vi "Configuration Utility.vi"() -> ()   [LabVIEW 2013, in "configuration library.lvlib"]
doc: "This is the main VI for the configuration editor."
uses:
  configuration library.lvlib
  Controls/StateCluster.ctl
  <vilib>/NI/Tag Bus Data Framework/Configuration Editor/Classes/SystemConfigRepo/SystemConfigRepo.lvclass
  <vilib>/CEF_TreeControl/Node/NodeRef.ctl
  <vilib>/CEF_TreeControl/Node/NISE_CEF_Node.lvclass
  <vilib>/CEF_TreeControl/Node/UserEventRef.ctl
  <vilib>/CEF_TreeControl/Controls/EventCluster.ctl
  subVI/SplashScreen/splash screen.ctl
  subVI/SplashScreen/notifier data.ctl
  Controls/add message.ctl
  Controls/MoveMessage.ctl
  <vilib>/NI/Tag Bus Module Framework/plugin discovery singleton/class discovery singleton methods.ctl
  <vilib>/NI/Tag Bus Data Framework/Configuration Editor/Classes/Systems/Systems.lvclass
  <vilib>/NI/Tag Bus Data Framework/Framework Configuration Classes/platypus configuration/systems cluster.ctl
  <vilib>/NI/Tag Bus Data Framework/Framework Configuration Classes/system configuration/PL_System Configuration.lvclass
  <vilib>/NI/Tag Bus Data Framework/Framework Configuration Classes/platypus configuration/targets cluster.ctl
  <vilib>/NI/Tag Bus Data Framework/Framework Configuration Classes/target configuration/PL_Target Configuration.lvclass
  <vilib>/NI/Tag Bus Data Framework/Framework Configuration Classes/platypus configuration/engines cluster.ctl
  <vilib>/NI/Module Execution Interface/Engine Configuration/engine configuration.lvclass
  <vilib>/NI/Tag Bus Module Framework/module configuration/TBM module configuration.lvclass
  <vilib>/NI/Tag Bus Data Framework/Configuration Editor/Classes/SystemConfigRepo/SystemConfigRepo.lvclass/SystemConfigRepo.ctl
  <vilib>/CEF_TreeControl/Repository/NISE_CEF_Repository.lvclass
  <vilib>/NI/AMC/Create Single Message.vi
  <vilib>/NI/AMC/Update Message Routing Info.vi
  <vilib>/NI/AMC/Read Termination Message.vi
  <vilib>/NI/Tag Bus Data Framework/Configuration Editor/subVIs/Glyphs Status.ctl
  <vilib>/NI/Tag Bus Data Framework/Configuration Editor/subVIs/Add status to name.vi
  <vilib>/NI/AMC/Send Message.vi
  <vilib>/NI/AMC/Globals.vi
  <vilib>/NI/Tag Bus Data Framework/Configuration Editor/Classes/Module editor node/module editor node.lvclass
  <vilib>/NI/Tag Bus Data Framework/Configuration Editor/Classes/EngineTags/EngineTags.lvclass
  <vilib>/NI/Module Timing Source/timing source/TBM timing source.lvclass
  <vilib>/NI/Tag Bus Data Framework/Configuration Editor/Classes/TBM Configuration Node/TBM Configuration Node.lvclass
  <vilib>/NI/Tag Bus Module Framework/root configuration/TBM configuration.lvclass
  <vilib>/NI/Tag Bus Data Framework/Configuration Editor/Classes/Targets/Targets.lvclass
  <vilib>/NI/Tag Bus Data Framework/Configuration Editor/Classes/Engine Parent/Engine Parent Editor Node.lvclass
  <vilib>/NI/Tag Bus Module Framework/channel/TBM channel.lvclass
  <vilib>/NI/AMC/AMC.lvlib
  <vilib>/CEF_TreeControl/NISE_CEF_TreeControl.lvlib
  subVI/SplashScreen/splash screen.lvlib
  <vilib>/NI/Tag Bus Data Framework/Framework Configuration Classes/class cache/PL_class cache.lvlib
  <vilib>/NI/Tag Bus Module Framework/plugin discovery singleton/class discovery singleton.lvlib
  <vilib>/NI/Tag Bus Data Framework/Configuration Editor/PL Framework Configuration Tool.lvlib
  <vilib>/NI/Tag Bus Data Framework/Framework Configuration Classes/platypus configuration/PLConfigurationSerializer.lvlib
panel:
  in  "Exit":bool
  in  "View":string(tree)
  # "Tag Bus Configuration Editor"
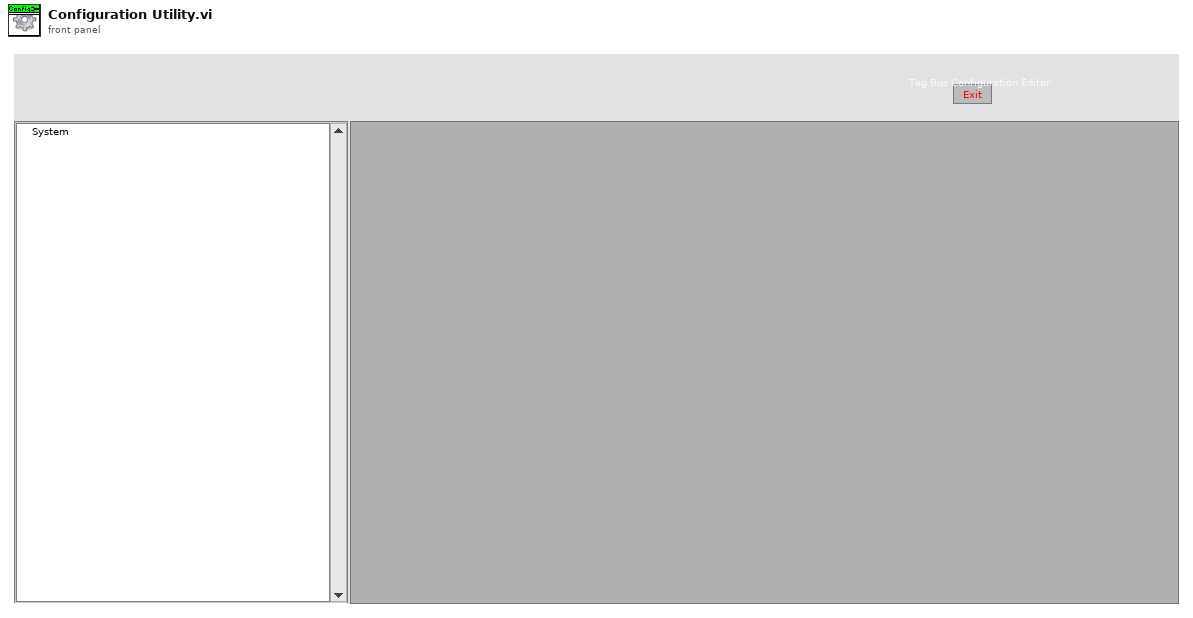
[diagram p1: front panel]
types:
  T1 = enum32{"Invalid", "Standard", "Closed", "Hidden", "Minimized", "Maximized"}
  T2 = typedef "configuration library.lvlib/StateCluster.ctl" = cluster{"repository":refnum<class "SystemConfigRepo.lvclass">, "root":T3, "unsaved changes":bool, "current path":path, "user event ref":T4, "glyph path":path[], "SplashScreen":T5, "classes cache":path}
  T3 = typedef "NISE_CEF_Node.lvclass/NodeRef.ctl" = refnum<data-value>
  T4 = typedef "NISE_CEF_Node.lvclass/UserEventRef.ctl" = refnum<user-event>
  T5 = typedef "configuration library.lvlib/splash screen.lvlib/splash screen.ctl" = cluster{"reference":refnum<vi>, "update notifier":refnum<notifier>, "Initialized":bool}
  T6 = typedef "AMC.lvlib/Message Queue.ctl" = refnum<queue>
  T7 = typedef "configuration library.lvlib/splash screen.lvlib/notifier data.ctl" = cluster{"Text":string, "percent":dbl}
  T8 = typedef "NISE_CEF_TreeControl.lvlib/EventCluster.ctl" = cluster{"command":string, "data":string}
  T9 = typedef "class discovery singleton.lvlib/class discovery singleton methods.ctl" = enum16{"add search paths", "load class by name", "list available classes", "get class path"}
  T10 = typedef "PLConfigurationSerializer.lvlib/systems cluster.ctl" = cluster{"System Configuration":refnum<class "PL_System Configuration.lvclass">, "targets":T11[]}
  T11 = typedef "PLConfigurationSerializer.lvlib/targets cluster.ctl" = cluster{"Target Configuration":refnum<class "PL_Target Configuration.lvclass">, "engines":T12[]}
  T12 = typedef "PLConfigurationSerializer.lvlib/engines cluster.ctl" = cluster{"engine configuration":refnum<class "engine configuration.lvclass">, "modules":refnum<class "TBM module configuration.lvclass">[]}
  T13 = cluster{"node id":string, "RightClickPath":string}
  T14 = typedef "configuration library.lvlib/add message.ctl" = cluster{"node type":string, "to add to":string}
  T15 = typedef "configuration library.lvlib/MoveMessage.ctl" = cluster{"node ref":T3, "new parent":T3}
  T16 = typedef "configuration library.lvlib/FilePaths.ctl" = cluster{"glyphs":path[], "classes":path, "classes cache":path}
  T17 = typedef "PL_class cache.lvlib/cache definition.ctl" = cluster{"configuration":T18, "class cache data":T19}
  T18 = typedef "PL_class cache.lvlib/cache search configuration.ctl" = cluster{"Search Paths":path[], "Folders to Exclude":string[], "full class list":path[]}
  T19 = typedef "PL_class cache.lvlib/cached class information.ctl" = cluster{"targets":T20[], "engines":T21[], "modules":T21[], "ignored class list":path[]}
  T20 = typedef "PL_class cache.lvlib/target class metadata.ctl" = cluster{"file name":string, "fully qualified name":string, "menu display name":string, "configuration class name":string}
  T21 = typedef "PL_class cache.lvlib/class metadata.ctl" = cluster{"file name":string, "fully qualified name":string, "menu display name":string, "configuration class":string, "instances allowed":i32, "supported targets":T22[]}
  T22 = typedef "TBM configuration.lvclass/Target Types.ctl" = enum16{"Windows", "Mac", "Linux", "Linux RT ARM", "VxWorks", "Pharlap", "Other", "Linux RT x64"}
  T23 = typedef "NISE_CEF_Node.lvclass/Summary.ctl" = cluster{"ID":string, "parent ID":string, "node type":string, "text":string, "additional text":string, "glyph":string, "depth":i32}
  T24 = typedef "LVPoint32TypeDef.ctl" = cluster{"Horizontal":i32, "Vertical":i32}
  T25 = cluster{"data name":string, "drag data":variant}[]
  T26 = typedef "NISE_CEF_Node.lvclass/NodeMenuOptions.ctl" = cluster{"removable":bool, "movable":bool, "duplicate":bool}
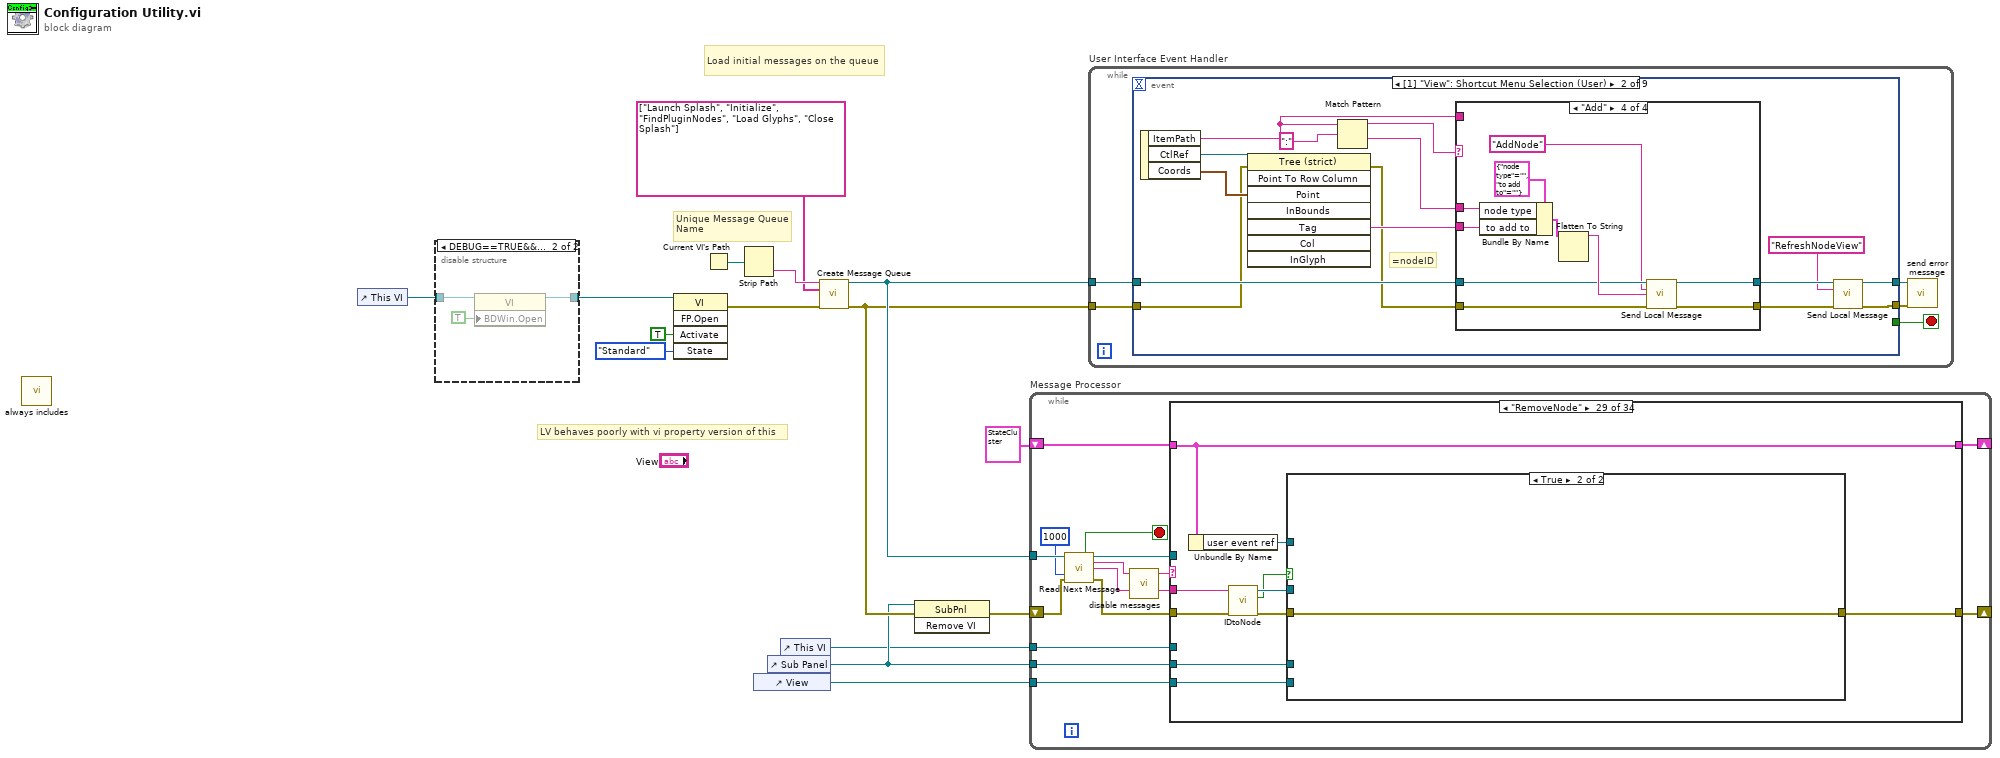
[diagram p0: block diagram]
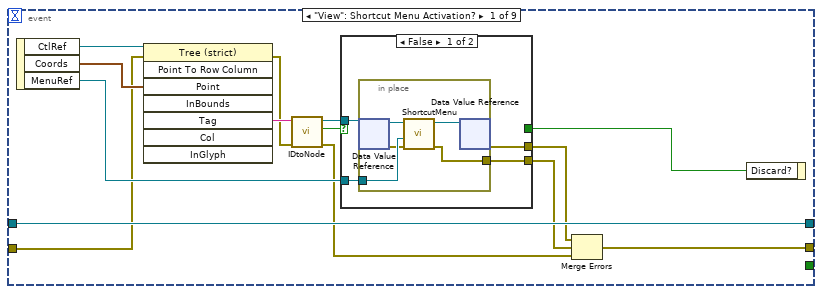
[diagram p3: hidden frame]
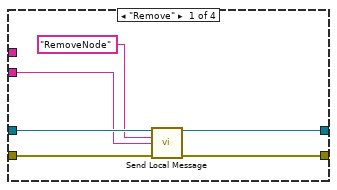
[diagram p5: hidden frame]
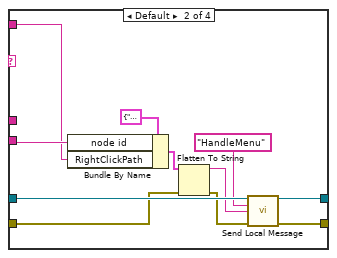
[diagram p6: hidden frame]
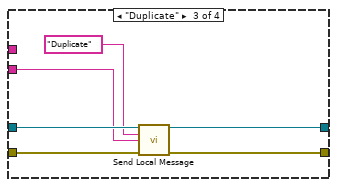
[diagram p7: hidden frame]
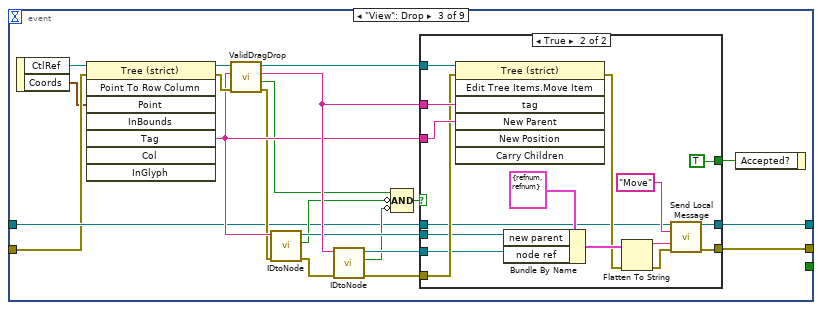
[diagram p8: hidden frame]
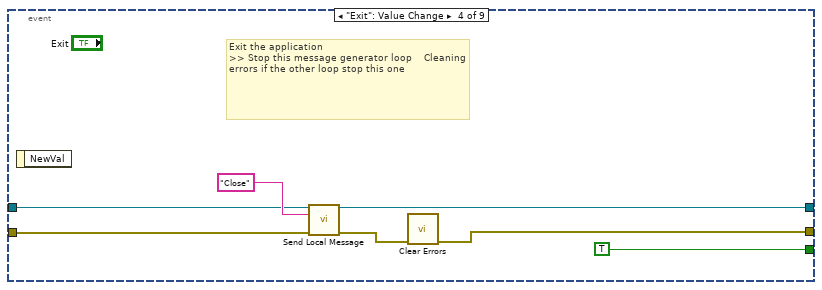
[diagram p10: hidden frame]
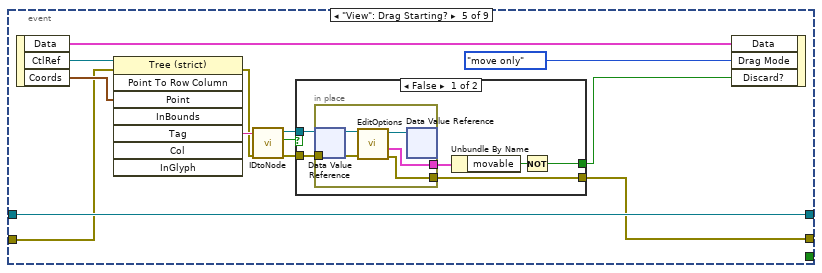
[diagram p11: hidden frame]
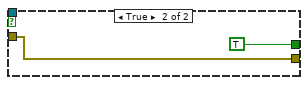
[diagram p12: hidden frame]
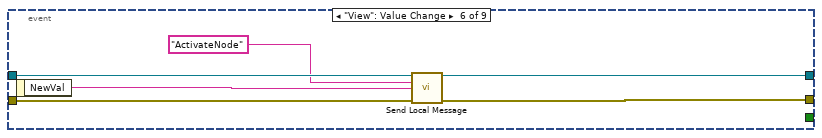
[diagram p13: hidden frame]
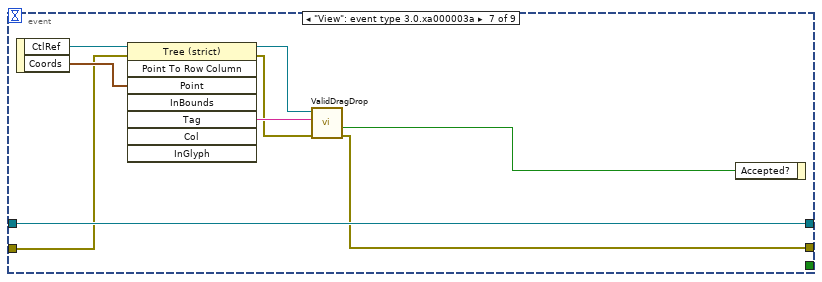
[diagram p14: hidden frame]
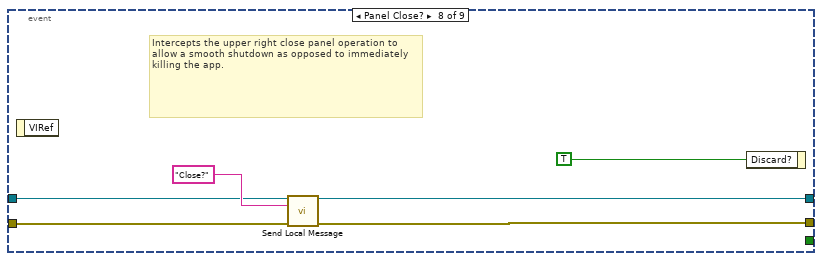
[diagram p15: hidden frame]
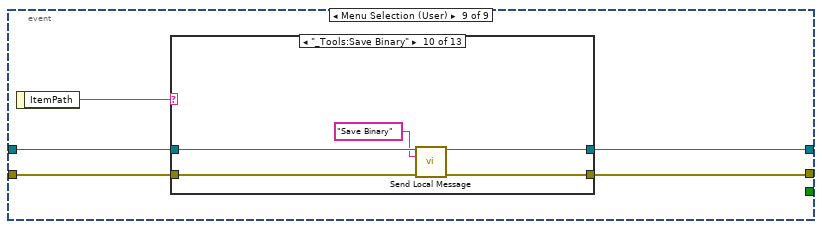
[diagram p16: hidden frame]
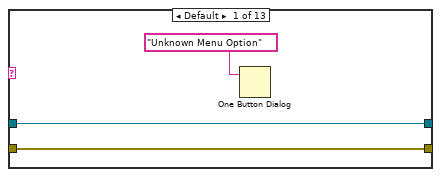
[diagram p17: hidden frame]
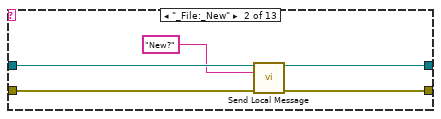
[diagram p18: hidden frame]
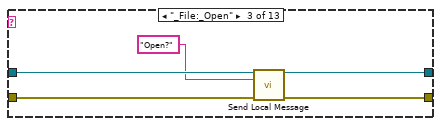
[diagram p19: hidden frame]
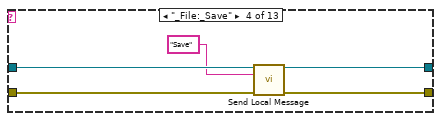
[diagram p20: hidden frame]
diagram:
  # "LV behaves poorly with vi property version of this"
  # "Unique Message Queue Name"
  # "Load initial messages on the queue"
  n1 = call "always includes.vi"() -> ()  [unwired: 12 in]
  n2 = control-ref of="This VI"() -> (w5:refnum<vi>)
  n3 = disable-structure shown="DEBUG==TRUE&&RUN_TIME_ENGINE==False" {
    disable-tunnel: [w16 w19] -> w6
    disable-tunnel: w5 -> [w16 w18]
    frame condition #0 (active) {
    }
    frame condition #1 {
      n4 = property class="VI"(reference=w18, "BDWin.Open"=TRUE ("Block Diagram Window:Open")) -> (reference out=w19:refnum<vi>)  [unwired: 1 in, 1 out]
    }
  }
  n5 = invoke class="VI" method="FP.Open"(reference=w6, "Activate"=TRUE ("Activate?"), "State"=T1."Standard") -> (error out=w9:errorcluster)  [unwired: 2 in, 4 out]
  n6 = Current VI's Path() -> (path=w14:path)
  n7 = Strip Path(path=w14) -> (name=w15:string)  [unwired: 1 out]
  n8 = control-ref of="View"() -> (w4:refnum<vi>)
  n9 = control-ref of="Sub Panel"() -> (w2:refnum<vi>)
  n10 = control-ref of="This VI"() -> (w1:refnum<vi>)
  n11 = call <vilib>:"Create Message Queue.vi"("message queue name"=w15, "initial message names"=string[] ["Launch Splash", "Initialize", "FindPluginNodes", "Load Glyphs", "Close Splash"], "error in"=w9) -> ("message queue out"=w12:T6, "error out"=w10:errorcluster)  [unwired: 11 in]
  n12 = invoke class="SubPnl" method="Remove VI"(reference=w2, error in=w10) -> (error out=w3:errorcluster)  [unwired: 1 in, 2 out]
  n13 = while "Message Processor" {
    shift-right: [w32] -> _
    shift-left: w3 -> [w31]
    tunnel: w12 -> [w30]
    shift-right: [w28] -> _
    shift-left: T2 {"repository"=refnum, "root"=refnum, "unsaved changes"=FALSE, "current path"=path "", "user event ref"=refnum, "glyph path"=[], "SplashScreen"={"reference"=refnum, "update notifier"=refnum, "Initialized"=FALSE}, "classes cache"=path ""} -> [w27]
    tunnel: w1 -> [w22]
    tunnel: w2 -> [w21]
    tunnel: w4 -> [w20]
    stop <- w34 stop-if-true
    n14 = call <vilib>:"Read Next Message.vi"("message queue in"=w30, "timeout (1 ms)"=1000, "error in"=w31) -> ("exit process?"=w34:bool, "message queue out"=w26:T6, "message name"=w23:string, "message value"=w25:string, "error out"=w33:errorcluster)  [unwired: 5 in, 3 out]
    n15 = call "disable messages.vi"("message to check"=w23) -> ("message out"=w24:string)  [unwired: 10 in]
    n16 = case shown="\"RemoveNode\"" w24 {
      selector: w24 -> [_ w38 _ _ _ _ _ _ _ _ _ w156 _ _ _ w278 _ _ _ _ _ _ _ _ _ _ _ _ _ _ _ _ _ _]
      tunnel: w25 -> [_ _ _ _ _ _ _ _ w112 _ _ _ _ _ _ _ _ w321 _ _ w383 _ w420 _ w458 w470 w488 _ w513 _ _ w560 w583 _]
      tunnel: w33 -> [w36 w41 w43 w50 w69 w76 w97 w103 w113 w139 w143 w153 w190 w202 w237 w270 w297 w326 w343 w348 w381 w395 w422 w437 w456 w469 w489 w501 w512 w538 w548 w559 w582 w588]
      tunnel: [w36 w41 w43 w53 w54 w83 w98 w106 errorcluster {"status"=FALSE, "code"=0, "source"=""} ("error out") w137 w143 w158 w193 w195 w230 w281 w308 w325 w342 w350 w368 w394 w413 w437 w457 w471 w492 w501 w511 w534 w545 w558 w581 w587] -> w32
      tunnel: [w35 w37 w42 w51 w56 w79 w88 w104 w114 w136 w142 w154 w191 w194 w229 w282 w309 w322 w344 w349 w384 w391 w421 w436 w439 w472 w490 w502 w505 w543 w547 w556 w584 w586] -> w28
      tunnel: w27 -> [w35 w37 w42 w52 w70 w79 w89 w104 w114 w136 w142 w155 w189 w203 w238 w277 w304 w323 w344 w349 w384 w392 w421 w436 w455 w472 w491 w503 w505 w543 w547 w556 w584 w586]
      tunnel: w26 -> [_ _ _ _ _ _ w99 w105 w116 w138 _ w157 w192 w201 w236 w267 w307 w324 _ w351 _ w393 w409 _ _ _ _ _ _ _ _ w557 w580 _]
      tunnel: w22 -> [_ _ _ w44 w62 _ w86 _ _ _ _ _ _ _ _ _ _ _ _ _ _ _ _ _ _ _ _ _ _ w533 _ _ _ _]
      tunnel: w21 -> [_ _ _ _ _ _ _ _ w107 w129 _ w145 _ _ _ w268 w295 _ _ _ _ _ _ _ _ _ _ _ w506 _ w544 w549 _ _]
      tunnel: w20 -> [_ _ _ _ _ w82 _ _ _ _ _ w144 _ _ _ _ _ _ _ _ _ _ w408 _ w440 w465 w483 _ w507 w537 _ _ _ _]
      frame "", "Idle" {
      }
      frame "Missing Message Handler", Default {
        # "Call this case if a message is received that is not handled by any other case. Typically this is a programming error as a result of a typo or unhandled message/missing message handler."
        n17 = Format Into String(format string="Internal Error: Missing message handler for '%s\" message." ("message"), w38) -> (resulting string=w40:string)  [unwired: 2 in, 1 out]
        n18 = One Button Dialog(message=w40) -> ()  [unwired: 2 out]
      }
      frame "------------Generic Operations------------" {
        # "Dummy case to add a seperation in the Case Structure menu"
      }
      frame "Launch Splash" {
        n19 = invoke class="VI" method="FP.Center"(reference=w44, error in=w50) -> (reference out=w48:refnum<vi>, error out=w47:errorcluster)  [unwired: 1 in, 1 out]
        n20 = invoke class="VI" method="FP.Open"(reference=w48, error in=w47, "State"=T1."Hidden") -> (error out=w45:errorcluster)  [unwired: 2 in, 4 out]
        n21 = call "Launch.vi"("error in"=w45) -> ("error out"=w53:errorcluster, "SplashScreen"=w49:T5)  [unwired: 9 in]
        n22 = Bundle By Name(cluster=w52, "SplashScreen"=w49) -> (w51:T2)
      }
      frame "Initialize" {
        # "issues in exe"
        n23 = Current VI's Menubar() -> (w68:refnum<k9>)
        n24 = call "menu options.vi"("error in"=w69, "VI ref"=w62, "menu ref in"=w68) -> ("error out"=w65:errorcluster)  [unwired: 7 in, 1 out]
        n25 = Create User Event(user event datatype=T8 {"command"="", "data"=""} ("Event"), error in=w65) -> (user event=w66:refnum<user-event>, error out=w54:errorcluster)
        n26 = call "default file paths.vi"() -> ("paths"=w67:T16)  [unwired: 11 in]
        n27 = Unbundle By Name(w67) -> ("classes cache"=w61:path, "glyphs"=w63:path[])
        n28 = Type Cast(type=T4 refnum ("user event ref"), x=w66) -> (*(type *) &x=w60:T4)
        n29 = Bundle By Name(cluster=w70, "user event ref"=w60, "classes cache"=w61, "glyph path"=w63) -> (w56:T2)
        n30 = Unbundle By Name(w56) -> ("SplashScreen"=w55:T5)
        n31 = call "Update.vi"("Update"=T7 {"Text"="Preparing UI...", "percent"=27.0}, "SplashScreen in"=w55) -> ("error out"=w58:errorcluster)  [unwired: 8 in, 1 out]
        n32 = call <vilib>:"Clear Errors.vi"("error in (no error)"=w58) -> ()  [unwired: 6 in, 1 out]
      }
      frame "Load Glyphs" {
        n33 = Unbundle By Name(w79) -> ("SplashScreen"=w78:T5, "glyph path"=w73:path[])
        n34 = call <vilib>:"class discovery singleton.vi"("error in"=w76, "method"=class_discovery_singleton_methods."list available classes") -> ("error out"=w72:errorcluster, "discovered classes"=w75:path[])  [unwired: 6 in, 2 out]
        n35 = for {
          tunnel: w75 -> [w85] mode=indexing
          tunnel: [w84] -> w74 mode=indexing
          n36 = Strip Path(path=w85) -> (stripped path=w84:path)  [unwired: 1 out]
        }
        n37 = Build Array (concatenate)(w73, w74) -> (w71:path[])
        n38 = call "Update.vi"("Update"=T7 {"Text"="Loading Glyphs...", "percent"=78.0}, "SplashScreen in"=w78) -> ("error out"=w81:errorcluster)  [unwired: 8 in, 1 out]
        n39 = call <vilib>:"Clear Errors.vi"("error in (no error)"=w81) -> ()  [unwired: 6 in, 1 out]
        n40 = call "Load Custom Status Glyph.vi"("tree ref"=w82, "error in"=w72, "glyph directories"=w71) -> ("error out"=w83:errorcluster)  [unwired: 8 in]
      }
      frame "Close Splash" {
        n41 = Unbundle By Name(w89) -> ("SplashScreen"=w95:T5)
        n42 = call "Close.vi"("error in"=w97, "SplashScreen"=w95) -> ("error out"=w91:errorcluster, "SplashScreen out"=w87:T5)  [unwired: 8 in]
        n43 = Bundle By Name(cluster=w89, "SplashScreen"=w87) -> (w88:T2)
        n44 = invoke class="VI" method="FP.Open"(reference=w86, error in=w91, "State"=T1."Standard") -> (reference out=w93:refnum<vi>, error out=w92:errorcluster)  [unwired: 2 in, 3 out]
        n45 = Close Reference(reference=w93, error in (no error)=w92) -> (error out=w90:errorcluster)
        n46 = call <vilib>:"Send Local Message.vi"("message queue in"=w99, "message name"="New" ("Message Name"), "error in"=w90) -> ("error out"=w98:errorcluster)  [unwired: 10 in, 2 out]
      }
      frame "Close" {
        n47 = Unbundle By Name(w104) -> ("root"=w101:T3)
        n48 = call <vilib>:"CloseNode.vi"("error in"=w103, "node ref"=w101) -> ("error out"=w100:errorcluster)  [unwired: 9 in]
        n49 = call <vilib>:"Send Local Message.vi"("message queue in"=w105, "message name"="Exit", "error in"=w100) -> ("error out"=w106:errorcluster)  [unwired: 10 in, 2 out]
      }
      frame "Error" {
        n50 = Unbundle By Name(w114) -> ("user event ref"=w110:T4)
        n51 = call "Remove UI without races.vi"("error in"=w113, "user event ref"=w110, "sub panel ref in"=w107) -> ("error out"=w108:errorcluster)  [unwired: 7 in, 1 out]
        n52 = case shown="\"\"" w112 {
          selector: w112 -> [w118 _]
          tunnel: w113 -> [w119 w120]
          tunnel: [w117 w120] -> w109
          frame Default {
            n53 = Unflatten From String(type=w119, binary string=w118, error in (no error)=w119) -> (value=w117:errorcluster)  [unwired: 2 in, 2 out]
          }
          frame "" {
          }
        }
        n54 = call <vilib>:"Clear Errors.vi"("error in (no error)"=w108) -> ()  [unwired: 6 in, 1 out]
        n55 = Unbundle By Name(w109) -> ("code"=w111:i32)
        n56 = case shown="15550" w111 {
          tunnel: w116 -> [_ _ _ w126 _]
          tunnel: w109 -> [_ _ _ w125 w128]
          frame -2147220623, -2147220621, -2147220364, 56, 63 {
            n57 = One Button Dialog(message="Problem communicating with remote device.  Make sure a valid device is selected and that the IP address is correct.") -> ()  [unwired: 1 in, 1 out]
          }
          frame 1003 {
            n58 = One Button Dialog(message="Dev Error: The Ui.vi for the selected class is broken") -> ()  [unwired: 1 in, 1 out]
          }
          frame 15550 {
            n59 = One Button Dialog(message="The cRIO does not yet have a configuration to download. Create or open a configuration and download it to the cRIO") -> ()  [unwired: 1 in, 1 out]
          }
          frame 537549 {
            n60 = call <vilib>:"Send Local Message.vi"("message queue in"=w126, "message name"="Exit", "error in"=w125) -> ()  [unwired: 10 in, 3 out]
            n61 = One Button Dialog(message="Invalid configuration file.") -> ()  [unwired: 1 in, 1 out]
          }
          frame 1, Default {
            n62 = call <vilib>:"Simple Error Handler.vi"("error in (no error)"=w128) -> ()  [unwired: 1 in, 8 out]
          }
        }
      }
      frame "Exit" {
        # "Stop the VI                                                                             >> Perform any cleanup tasks in this message case. >> Clear display before closing."
        n63 = call <vilib>:"Destroy Message Queue.vi"("message queue in"=w138, "error in"=w139) -> ("error out"=w133:errorcluster)  [unwired: 11 in, 2 out]
        n64 = control-ref of="Exit"() -> (w135:refnum<vi>)
        n65 = Unbundle By Name(w136) -> ("user event ref"=w130:T4)
        n66 = property class="Bool (strict)"(reference=w135, error in=w133, "Val(Sgnl)"=FALSE ("Exit")) -> (error out=w132:errorcluster)  [unwired: 1 out]
        n67 = call "Remove UI without races.vi"("error in"=w132, "user event ref"=w130, "sub panel ref in"=w129) -> ("error out"=w131:errorcluster)  [unwired: 7 in, 1 out]
        n68 = disable-structure shown="RUN_TIME_ENGINE==True" {
          disable-tunnel: [w140 w141] -> w137
          disable-tunnel: w131 -> [w140 w141]
          frame condition #0 (active) {
          }
          frame condition #1 {
            n69 = Quit LabVIEW() -> ()  [unwired: 1 in]
          }
        }
      }
      frame "------------Menu Operations--------------" {
        # "Dummy case to add a seperation in the Case Structure menu"
      }
      frame "Close?", "New?", "Open?" {
        n70 = Unbundle By Name(w155) -> ("unsaved changes"=w146:bool, "user event ref"=w147:T4)
        n71 = case shown="True" w146 {
          tunnel: [TRUE ("SaveFlag") w176] -> w149
          tunnel: w155 -> [w168 w175]
          tunnel: [w168 w174] -> w154
          tunnel: w153 -> [w167 w173]
          tunnel: [w167 w172] -> w148
          tunnel: w145 -> [_ w171]
          tunnel: w144 -> [_ w170]
          frame False {
            # "If there is nothing to save Go do Action"
          }
          frame True {
            n72 = call "dialog save dirty dot.vi"("error in"=w173, "View"=w170, "sub panel ref in"=w171, "state in"=w175) -> ("error out"=w172:errorcluster, "new"=w176:bool, "state out"=w174:T2)  [unwired: 5 in]
          }
        }
        n73 = Search and Replace String(input string=w156, search string="?", replace string="") -> (result string=w150:string)  [unwired: 5 in, 3 out]
        n74 = case shown="True" w149 {
          tunnel: w148 -> [w159 w166]
          tunnel: [w159 w162] -> w158
          tunnel: w157 -> [_ w165]
          tunnel: w150 -> [_ w164]
          tunnel: w147 -> [_ w161]
          tunnel: w145 -> [_ w160]
          frame False {
          }
          frame True {
            n75 = call <vilib>:"Send Local Message.vi"("message queue in"=w165, "message name"=w164, "error in"=w166) -> ("error out"=w163:errorcluster)  [unwired: 10 in, 2 out]
            n76 = call "Remove UI without races.vi"("error in"=w163, "user event ref"=w161, "sub panel ref in"=w160) -> ("error out"=w162:errorcluster)  [unwired: 7 in, 1 out]
          }
        }
      }
      frame "New" {
        # "unused"
        n77 = call <vilib>:"create default cache.vi"() -> ("cache"=w179:T17)  [unwired: 11 in]
        n78 = Unbundle By Name(w179) -> ("configuration.Search Paths"=w178:path[])
        n79 = call-dynamic "Initialize.vi"("error in"=w190, "node in"=refnum<class "Systems.lvclass"> refnum ("Systems.lvclass")) -> ("error out"=w185:errorcluster, "data value reference"=w186:T3)  [unwired: 7 in, 1 out]
        n80 = Delete From Array(array=w178) -> (deleted portion=w177:path)  [unwired: 2 in, 1 out]
        n81 = call-dynamic "Initialize.vi"("error in"=w185, "path"=w177, "repository in"=refnum<class "SystemConfigRepo.lvclass"> refnum ("SystemConfigRepo.lvclass")) -> ("error out"=w184:errorcluster, "repository out"=w183:refnum<class "SystemConfigRepo.lvclass">)  [unwired: 7 in]
        n82 = Bundle By Name(cluster=w189, "unsaved changes"=FALSE ("SaveFlag"), "repository"=w183, "root"=w186, "current path"=path "") -> (w191:T2)
        n83 = call <vilib>:"Send Local Message.vi"("message queue in"=w192, "message name"="PopulateTree", "error in"=w184) -> ("error out"=w193:errorcluster)  [unwired: 10 in, 2 out]
      }
      frame "Open" {
        n84 = call <vilib>:"Set Busy.vi"() -> ("error out"=w198:errorcluster)  [unwired: 10 in, 1 out]
        n85 = call "File Dialog"("pattern (all files)"="*.pcfg") -> ("selected path"=w200:path, "cancelled"=w199:bool)  [unwired: 11 in, 2 out]
        n86 = case shown="False" w199 {
          tunnel: w203 -> [w212 w228]
          tunnel: [w211 w228] -> w194
          tunnel: w202 -> [w210 w227]
          tunnel: w201 -> [w209 _]
          tunnel: [w208 w227] -> w195
          tunnel: w200 -> [w205 _]
          tunnel: w198 -> [w204 w226]
          tunnel: [w204 w226] -> w197
          frame False {
            n87 = in-place {
              in-place-border: w210 -> [w225]
              in-place-border: [w214] -> w206
              in-place-border: w205 -> [w220]
              n88 = in-place-cluster #1(w212) -> ("repository"=w213:refnum<class "SystemConfigRepo.lvclass">, "current path"=w221:path)  [unwired: 2 out]
              n89 = call-dynamic "Open.vi"("error in"=w225, "file path"=w220, "SystemConfigRepo in"=w213) -> ("error out"=w222:errorcluster, "SystemConfigRepo out"=w218:refnum<class "SystemConfigRepo.lvclass">)  [unwired: 6 in, 1 out]
              n90 = call-dynamic "WriteTree.vi"("error in"=w222, "SystemConfigRepo in"=w218) -> ("error out"=w215:errorcluster, "root"=w223:T3, "repository out"=w217:refnum<class "NISE_CEF_Repository.lvclass">)  [unwired: 7 in]
              n91 = To More Specific Class(target class=w213, reference=w217, error in=w215) -> (specific class reference=w216:refnum<class "SystemConfigRepo.lvclass">, error out=w214:errorcluster)
              n92 = Select(t=w221, s=w214, f=w220) -> (s? t:f=w219:path)
              n93 = in-place-cluster #1("unsaved changes"=FALSE ("SaveFlag"), "repository"=w216, "root"=w223, "current path"=w219) -> (w211:T2)
            }
            n94 = call <vilib>:"Send Local Message.vi"("message queue in"=w209, "message name"="PopulateTree", "error in"=w206) -> ("error out"=w208:errorcluster)  [unwired: 10 in, 2 out]
          }
          frame True {
          }
        }
        n95 = call <vilib>:"Unset Busy.vi"("error in (no error)"=w197) -> ()  [unwired: 10 in, 1 out]
      }
      frame "Load Binary" {
        n96 = call <vilib>:"Set Busy.vi"() -> ("error out"=w233:errorcluster)  [unwired: 10 in, 1 out]
        n97 = call "File Dialog2"("pattern (all files)"="*.pbin") -> ("selected path"=w235:path, "cancelled"=w234:bool)  [unwired: 11 in, 2 out]
        n98 = case shown="False" w234 {
          tunnel: w238 -> [w247 w266]
          tunnel: [w246 w266] -> w229
          tunnel: w237 -> [w245 w265]
          tunnel: w236 -> [w244 _]
          tunnel: [w243 w265] -> w230
          tunnel: w235 -> [w240 _]
          tunnel: w233 -> [w239 w264]
          tunnel: [w239 w264] -> w232
          frame False {
            n99 = in-place {
              in-place-border: w245 -> [w254]
              in-place-border: [w258] -> w241
              in-place-border: w240 -> [w250]
              n100 = in-place-cluster #2(w247) -> ("repository"=w256:refnum<class "SystemConfigRepo.lvclass">)  [unwired: 2 out]
              n101 = Read from Binary File(5:T10 {"System Configuration"=refnum, "targets"=[]} ("system"), 8:w254, 11:w250) -> (0:w253:errorcluster, 2:w251:T10, 3:w248:refnum<file>)  [unwired: 3 in, 1 out]
              n102 = Close File(refnum=w248, error in=w253) -> (error out=w249:errorcluster)  [unwired: 1 out]
              n103 = call <vilib>:"Write Systems.vi"("error in"=w249, "system"=w251, "SystemConfigRepo in"=w256) -> ("error out"=w255:errorcluster, "SystemConfigRepo out"=w257:refnum<class "SystemConfigRepo.lvclass">)  [unwired: 7 in]
              n104 = call-dynamic "WriteTree.vi"("error in"=w255, "SystemConfigRepo in"=w257) -> ("error out"=w259:errorcluster, "root"=w262:T3, "repository out"=w261:refnum<class "NISE_CEF_Repository.lvclass">)  [unwired: 7 in]
              n105 = To More Specific Class(target class=w256, reference=w261, error in=w259) -> (specific class reference=w260:refnum<class "SystemConfigRepo.lvclass">, error out=w258:errorcluster)
              n106 = in-place-cluster #2("unsaved changes"=TRUE ("SaveFlag"), "repository"=w260, "root"=w262) -> (w246:T2)
            }
            n107 = call <vilib>:"Send Local Message.vi"("message queue in"=w244, "message name"="PopulateTree", "error in"=w241) -> ("error out"=w243:errorcluster)  [unwired: 10 in, 2 out]
          }
          frame True {
          }
        }
        n108 = call <vilib>:"Unset Busy.vi"("error in (no error)"=w232) -> ()  [unwired: 10 in, 1 out]
      }
      frame "Save", "SaveAs" {
        n109 = Unbundle By Name(w277) -> ("user event ref"=w271:T4)
        n110 = call <vilib>:"Set Busy.vi"() -> ("error out"=w275:errorcluster)  [unwired: 10 in, 1 out]
        n111 = call "Remove UI without races.vi"("error in"=w270, "user event ref"=w271, "sub panel ref in"=w268) -> ("error out"=w269:errorcluster)  [unwired: 7 in, 1 out]
        n112 = flat-sequence {
          tunnel: w269 -> [w289]
          tunnel: w278 -> [w287]
          tunnel: w277 -> [w284]
          tunnel: w275 -> [w283]
          tunnel: [w290] -> w274
          tunnel: [w288] -> w273
          tunnel: [w283] -> w272
          tunnel: [w292] -> w276
          tunnel: [w293] -> w279
          tunnel: [w294] -> w282
          tunnel: w274 -> [w294]
          tunnel: w273 -> [w293]
          tunnel: w272 -> [w292]
          frame #0 {
            n113 = Equal?(x="SaveAs", y=w287) -> (x = y?=w286:bool)
            n114 = call "save operation.vi"("force save as"=w286, "error in"=w289, "state cluster"=w284) -> ("error out"=w288:errorcluster, "state out"=w290:T2)  [unwired: 7 in]
          }
          frame #1 {
            n115 = local read "View"() -> (w291:string)
            n116 = property on="View" class="Tree (strict)"("Val(Sgnl)"=w291) -> ()  [unwired: 2 in, 2 out]
          }
        }
        n117 = call <vilib>:"Unset Busy.vi"("error in (no error)"=w276) -> ()  [unwired: 10 in, 1 out]
        n118 = call <vilib>:"Send Local Message.vi"("message queue in"=w267, "message name"="PopulateTree", "error in"=w279) -> ("error out"=w281:errorcluster)  [unwired: 10 in, 2 out]
      }
      frame "Save Binary" {
        n119 = Unbundle By Name(w304) -> ("user event ref"=w298:T4)
        n120 = call <vilib>:"Set Busy.vi"() -> ("error out"=w302:errorcluster)  [unwired: 10 in, 1 out]
        n121 = call "Remove UI without races.vi"("error in"=w297, "user event ref"=w298, "sub panel ref in"=w295) -> ("error out"=w296:errorcluster)  [unwired: 7 in, 1 out]
        n122 = flat-sequence {
          tunnel: w296 -> [w313]
          tunnel: w304 -> [w310]
          tunnel: w302 -> [w314]
          tunnel: [w311] -> w301
          tunnel: [w312] -> w300
          tunnel: [w314] -> w299
          tunnel: [w316] -> w303
          tunnel: [w317] -> w305
          tunnel: [w318] -> w309
          tunnel: w301 -> [w318]
          tunnel: w300 -> [w317]
          tunnel: w299 -> [w316]
          frame #0 {
            n123 = call "save operation binary.vi"("error in"=w313, "state cluster"=w310) -> ("error out"=w312:errorcluster, "state out"=w311:T2)  [unwired: 8 in]
          }
          frame #1 {
            n124 = local read "View"() -> (w315:string)
            n125 = property on="View" class="Tree (strict)"("Val(Sgnl)"=w315) -> ()  [unwired: 2 in, 2 out]
          }
        }
        n126 = call <vilib>:"Unset Busy.vi"("error in (no error)"=w303) -> ()  [unwired: 10 in, 1 out]
        n127 = call <vilib>:"Send Local Message.vi"("message queue in"=w307, "message name"="PopulateTree", "error in"=w305) -> ("error out"=w308:errorcluster)  [unwired: 10 in, 2 out]
      }
      frame "Custom View" {
        n128 = in-place {
          in-place-border: w326 -> [w339]
          in-place-border: [w330] -> w319
          in-place-border: w321 -> [w331]
          n129 = in-place-cluster #3(w323) -> ("repository"=w328:refnum<class "SystemConfigRepo.lvclass">, "root"=w337:T3)
          n130 = call-dynamic "ReadTree.vi"("error in"=w339, "root"=w337, "SystemConfigRepo in"=w328) -> ("error out"=w335:errorcluster, "repository out"=w333:refnum<class "NISE_CEF_Repository.lvclass">)  [unwired: 7 in]
          n131 = call-dynamic "CustomView.vi"("error in"=w335, "view name"=w331, "repository in"=w333) -> ("error out"=w334:errorcluster, "repository out"=w332:refnum<class "NISE_CEF_Repository.lvclass">)  [unwired: 7 in]
          n132 = call-dynamic "WriteTree.vi"("error in"=w334, "repository in"=w332) -> ("error out"=w338:errorcluster, "root"=w336:T3, "repository out"=w329:refnum<class "NISE_CEF_Repository.lvclass">)  [unwired: 7 in]
          n133 = To More Specific Class(target class=w328, reference=w329, error in=w338) -> (specific class reference=w327:refnum<class "SystemConfigRepo.lvclass">, error out=w330:errorcluster)
          n134 = in-place-cluster #3("repository"=w327, "root"=w336) -> (w322:T2)
        }
        n135 = call <vilib>:"Send Local Message.vi"("message queue in"=w324, "message name"="PopulateTree", "error in"=w319) -> ("error out"=w325:errorcluster)  [unwired: 10 in, 2 out]
      }
      frame "DeployTool" {
        n136 = Unbundle By Name(w344) -> ("current path"=w340:path, "root"=w341:T3)
        n137 = call <vilib>:"deployment tool.vi"("current pcfg path"=w340, "error in"=w343, "node ref"=w341) -> ("error out"=w342:errorcluster)  [unwired: 8 in]
      }
      frame "Edit Plugin Search Paths" {
        n138 = Unbundle By Name(w349) -> ("classes cache"=w345:path)
        n139 = call <vilib>:"load cache.vi"("error in"=w348, "cache path"=w345) -> ("error out"=w346:errorcluster, "cache"=w347:T17)  [unwired: 8 in]
        n140 = Unbundle By Name(w347) -> ("configuration.Search Paths"=w355:path[])
        n141 = call "dialog edit search paths.vi"("error in"=w346, "Plugin Search Paths"=w355) -> ("error out"=w352:errorcluster, "Cancelled?"=w354:bool, "Plugin Search Paths"=w353:path[])  [unwired: 7 in]
        n142 = case shown="False" w354 {
          tunnel: w347 -> [w365 _]
          tunnel: w353 -> [w364 _]
          tunnel: w352 -> [w358 w366]
          tunnel: w351 -> [w361 _]
          tunnel: [w360 w366] -> w350
          tunnel: w345 -> [w356 _]
          frame False {
            n143 = Bundle By Name(cluster=w365, "configuration.Search Paths"=w364) -> (w357:T17)
            n144 = call <vilib>:"save cache.vi"("error in"=w358, "cache"=w357, "path"=w356) -> ("error out"=w359:errorcluster)  [unwired: 8 in]
            n145 = call <vilib>:"Send Local Message.vi"("message queue in"=w361, "message name"="FindPluginNodes", "message value"="Refresh", "error in"=w359) -> ("error out"=w360:errorcluster)  [unwired: 9 in, 2 out]
          }
          frame True {
          }
        }
      }
      frame "FindPluginNodes" {
        n146 = call <vilib>:"Set Busy.vi"("error in (no error)"=w381) -> ("error out"=w380:errorcluster)  [unwired: 9 in, 1 out]
        n147 = Unbundle By Name(w384) -> ("SplashScreen"=w374:T5, "classes cache"=w370:path)
        n148 = Equal?(x="Refresh", y=w383) -> (x = y?=w375:bool)
        n149 = call <vilib>:"load cache.vi"("error in"=w380, "cache path"=w370) -> ("error out"=w379:errorcluster, "cache"=w378:T17)  [unwired: 8 in]
        n150 = case shown="Error" w379 {
          selector: w379 -> [w387 _]
          tunnel: [w385 w388] -> w376
          tunnel: w378 -> [w386 _]
          tunnel: [w387 _] -> w377
          frame No Error {
            n151 = call <vilib>:"remove missing files.vi"("cache in"=w386) -> ("cache out"=w385:T17)  [unwired: 10 in]
          }
          frame Error {
            n152 = call <vilib>:"create default cache.vi"() -> ("cache"=w388:T17)  [unwired: 11 in]
          }
        }
        n153 = call <vilib>:"identify new classes.vi"("error in"=w377, "force scan"=w375, "cache in"=w376) -> ("error out"=w371:errorcluster, "cache out"=w367:T17)  [unwired: 7 in]
        n154 = call "Update.vi"("Update"=T7 {"Text"="Loading Classes...", "percent"=45.0}, "SplashScreen in"=w374) -> ("error out"=w373:errorcluster)  [unwired: 8 in, 1 out]
        n155 = call <vilib>:"Clear Errors.vi"("error in (no error)"=w373) -> ()  [unwired: 6 in, 1 out]
        n156 = call <vilib>:"save cache.vi"("error in"=w371, "cache"=w367, "path"=w370) -> ("error out"=w369:errorcluster)  [unwired: 8 in]
        n157 = call <vilib>:"Unset Busy.vi"("error in (no error)"=w369) -> ("error out"=w368:errorcluster)  [unwired: 10 in]
      }
      frame "Test" {
        n158 = in-place {
          in-place-border: w395 -> [w407]
          in-place-border: [w402] -> w389
          n159 = in-place-cluster #4(w392) -> ("repository"=w397:refnum<class "SystemConfigRepo.lvclass">, "root"=w404:T3)
          n160 = call-dynamic "ReadTree.vi"("error in"=w407, "root"=w404, "SystemConfigRepo in"=w397) -> ("error out"=w403:errorcluster, "repository out"=w399:refnum<class "NISE_CEF_Repository.lvclass">)  [unwired: 7 in]
          n161 = To More Specific Class(target class=w397, reference=w399, error in=w403) -> (specific class reference=w398:refnum<class "SystemConfigRepo.lvclass">, error out=w400:errorcluster)
          n162 = call-dynamic "WriteTree.vi"("error in"=w400, "SystemConfigRepo in"=w398) -> ("error out"=w406:errorcluster, "root"=w405:T3, "repository out"=w401:refnum<class "NISE_CEF_Repository.lvclass">)  [unwired: 7 in]
          n163 = To More Specific Class(target class=w397, reference=w401, error in=w406) -> (specific class reference=w396:refnum<class "SystemConfigRepo.lvclass">, error out=w402:errorcluster)
          n164 = in-place-cluster #4("repository"=w396, "root"=w405) -> (w391:T2)
        }
        n165 = call <vilib>:"Send Local Message.vi"("message queue in"=w393, "message name"="PopulateTree", "error in"=w389) -> ("error out"=w394:errorcluster)  [unwired: 10 in, 2 out]
      }
      frame "HandleMenu" {
        n166 = Unflatten From String(type=T13 {"node id"="", "RightClickPath"=""} ("input cluster"), binary string=w420, error in (no error)=w422) -> (value=w418:T13, error out=w417:errorcluster)  [unwired: 2 in, 1 out]
        n167 = Unbundle By Name(w418) -> ("RightClickPath"=w411:string, "node id"=w416:string)
        n168 = call <vilib>:"IDtoNode.vi"("error in"=w417, "ID"=w416) -> ("error out"=w414:errorcluster, "node ref"=w415:T3)  [unwired: 7 in, 1 out]
        n169 = in-place {
          in-place-border: w414 -> [w435]
          in-place-border: [w430] -> w413
          in-place-border: [w429] -> w412
          in-place-border: w411 -> [w428]
          in-place-border: [w428] -> w410
          in-place-border: w409 -> [w427]
          in-place-border: w408 -> [w426]
          n170 = in-place-dvr #5(w415) -> (w432:refnum<class "NISE_CEF_Node.lvclass">, w434:errorcluster)
          n171 = Merge Errors(w435, w434) -> (w433:errorcluster)
          n172 = call-dynamic "MenuHandler.vi"("tree control"=w426, "message queue out"=w427, "error in (no error)"=w433, "menu string"=w428, "NISE_CEF_Node in"=w432) -> ("error out"=w430:errorcluster, "Unhandled"=w429:bool, "NISE_CEF_Node out"=w431:refnum<class "NISE_CEF_Node.lvclass">)  [unwired: 4 in]
          n173 = in-place-dvr #5(w431) -> ()  [unwired: 2 out]
        }
        n174 = case shown="True" w412 {
          tunnel: w410 -> [_ w423]
          frame False {
          }
          frame True {
            n175 = Concatenate Strings("Unknown item path:\n" ("message"), w423) -> (w425:string)
            n176 = One Button Dialog(message=w425) -> ()  [unwired: 1 in, 1 out]
          }
        }
      }
      frame "-------TreeControl Operations-----------" {
        # "Dummy case to add a seperation in the Case Structure menu"
      }
      frame "AddNode" {
        n177 = call <vilib>:"Set Busy.vi"("error in (no error)"=w456) -> ("error out"=w441:errorcluster)  [unwired: 9 in, 1 out]
        n178 = Unflatten From String(type=T14 {"node type"="", "to add to"=""} ("input cluster"), binary string=w458) -> (value=w451:T14)  [unwired: 3 in, 2 out]
        n179 = Unbundle By Name(w451) -> ("to add to"=w448:string, "node type"=w444:string)
        n180 = in-place {
          in-place-border: w444 -> [w464]
          in-place-border: [w461] -> w443
          in-place-border: w441 -> [w460]
          in-place-border: [w459] -> w442
          n181 = in-place-cluster #6(w455) -> ("repository"=w463:refnum<class "SystemConfigRepo.lvclass">)
          n182 = call-dynamic "GetClassPath.vi"("error in"=w460, "class name"=w464, "SystemConfigRepo in"=w463) -> ("error out"=w459:errorcluster, "class path"=w461:path, "SystemConfigRepo out"=w462:refnum<class "SystemConfigRepo.lvclass">)  [unwired: 6 in]
          n183 = in-place-cluster #6("repository"=w462) -> (w439:T2)
        }
        n184 = call <vilib>:"Get LV Class Default Value.vi"("error in (no error)"=w442, "class path"=w443) -> ("error out"=w453:errorcluster, "object"=w454:refnum<class>)  [unwired: 8 in]
        n185 = To More Specific Class(target class=refnum<class "NISE_CEF_Node.lvclass"> refnum ("NISE_CEF_Node.lvclass"), reference=w454, error in=w453) -> (specific class reference=w450:refnum<class "NISE_CEF_Node.lvclass">, error out=w447:errorcluster)
        n186 = call <vilib>:"AddNode.vi"("error in"=w447, "node in"=w450, "parent node ID"=w448) -> ("error out"=w446:errorcluster, "summary"=w445:T23[])  [unwired: 7 in]
        n187 = call <vilib>:"PopulateTreeSumary.vi"("error in"=w446, "array"=w445, "tree ref in"=w440) -> ("error out"=w438:errorcluster)  [unwired: 8 in]
        n188 = call <vilib>:"Unset Busy.vi"("error in (no error)"=w438) -> ("error out"=w457:errorcluster)  [unwired: 10 in]
      }
      frame "Duplicate" {
        n189 = call <vilib>:"IDtoNode.vi"("error in"=w469, "ID"=w470) -> ("error out"=w467:errorcluster, "invalid Id"=w466:bool, "node ref"=w468:T3)  [unwired: 7 in]
        n190 = case shown="False" w466 {
          tunnel: [w481 w482] -> w471
          tunnel: w468 -> [w480 _]
          tunnel: w467 -> [w477 w482]
          tunnel: w465 -> [w473 _]
          frame False {
            n191 = call <vilib>:"DuplicateNode.vi"("same parent?"=TRUE ("s"), "error in"=w477, "node ref in"=w480) -> ("error out"=w478:errorcluster, "new node ref"=w479:T3)  [unwired: 7 in]
            n192 = call <vilib>:"Summary.vi"("error in"=w478, "node self ref"=w479) -> ("error out"=w475:errorcluster, "summary"=w474:T23[])  [unwired: 8 in]
            n193 = call <vilib>:"PopulateTreeSumary.vi"("error in"=w475, "array"=w474, "tree ref in"=w473) -> ("error out"=w481:errorcluster)  [unwired: 8 in]
          }
          frame True {
          }
        }
      }
      frame "RefreshNode" {
        # "Refreshes the node in the Tree               Sets the save flag to true                       This case can be called from the UIs of the nodes"
        n194 = call <vilib>:"IDtoNode.vi"("error in"=w489, "ID"=w488) -> ("error out"=w486:errorcluster, "invalid Id"=w484:bool, "node ref"=w485:T3)  [unwired: 7 in]
        n195 = case shown="False" w484 {
          tunnel: [w498 w499] -> w492
          tunnel: w486 -> [w495 w499]
          tunnel: w485 -> [w494 _]
          tunnel: w483 -> [w493 _]
          frame False {
            n196 = call <vilib>:"Summary.vi"("error in"=w495, "node self ref"=w494) -> ("error out"=w497:errorcluster, "summary"=w496:T23[])  [unwired: 8 in]
            n197 = call <vilib>:"RefreshSubTree.vi"("error in"=w497, "node information"=w496, "tree ref in"=w493) -> ("error out"=w498:errorcluster)  [unwired: 7 in, 1 out]
          }
          frame True {
          }
        }
        n198 = Bundle By Name(cluster=w491, "unsaved changes"=TRUE ("SaveFlag")) -> (w490:T2)
      }
      frame "SetDirtyDot" {
        n199 = Bundle By Name(cluster=w503, "unsaved changes"=TRUE ("SaveFlag")) -> (w502:T2)
      }
      frame "RemoveNode" {
        n200 = Unbundle By Name(w505) -> ("user event ref"=w504:T4)
        n201 = call <vilib>:"IDtoNode.vi"("error in"=w512, "ID"=w513) -> ("error out"=w510:errorcluster, "invalid Id"=w508:bool, "node ref"=w509:T3)  [unwired: 7 in]
        n202 = case shown="True" w508 {
          tunnel: w510 -> [w521 w531]
          tunnel: w509 -> [w519 _]
          tunnel: [w523 w531] -> w511
          tunnel: w507 -> [w522 _]
          tunnel: w506 -> [w518 _]
          tunnel: w504 -> [w517 _]
          frame False {
            n203 = call "check if subpanel should be closed.vi"("error in"=w521, "SubPanel in"=w518, "node in"=w519) -> ("error out"=w516:errorcluster, "needs closing"=w514:bool, "node out"=w520:T3)  [unwired: 6 in]
            n204 = case shown="True" w514 {
              tunnel: w518 -> [_ w530]
              tunnel: w517 -> [_ w529]
              tunnel: w516 -> [w526 w528]
              tunnel: [w526 w527] -> w515
              frame False {
              }
              frame True {
                n205 = call "Remove UI without races.vi"("error in"=w528, "user event ref"=w529, "sub panel ref in"=w530) -> ("error out"=w527:errorcluster)  [unwired: 7 in, 1 out]
              }
            }
            n206 = call <vilib>:"RemoveNode.vi"("error in"=w515, "node"=w520) -> ("error out"=w524:errorcluster, "node ID"=w525:string)  [unwired: 8 in]
            n207 = call <vilib>:"ClearTreeNode.vi"("error in"=w524, "tag"=w525, "tree reference"=w522) -> ("error out"=w523:errorcluster)  [unwired: 8 in]
          }
          frame True {
          }
        }
      }
      frame "PopulateTree" {
        n208 = Unbundle By Name(w543) -> ("current path"=w536:path, "root"=w540:T3)
        n209 = call <vilib>:"Summary.vi"("error in"=w538, "depth"=0 ("Depth"), "node self ref"=w540) -> ("error out"=w541:errorcluster, "summary"=w542:T23[])  [unwired: 7 in]
        n210 = Strip Path(path=w536) -> (name=w532:string)  [unwired: 1 out]
        n211 = call <vilib>:"RefreshEntireTree.vi"("calling VI in"=w533, "error in"=w541, "array"=w542, "tree ref in"=w537) -> ("error out"=w535:errorcluster)  [unwired: 7 in]
        n212 = property class="VI"(reference=w533, error in=w535, "Front Panel.Title"=w532) -> (error out=w534:errorcluster)  [unwired: 1 out]
      }
      frame "CleansubPanel" {
        n213 = Unbundle By Name(w547) -> ("user event ref"=w546:T4)
        n214 = call "Remove UI without races.vi"("error in"=w548, "user event ref"=w546, "sub panel ref in"=w544) -> ("error out"=w545:errorcluster)  [unwired: 7 in, 1 out]
      }
      frame "ActivateNode" {
        n215 = Unbundle By Name(w556) -> ("user event ref"=w553:T4)
        n216 = call <vilib>:"Set Busy.vi"("error in (no error)"=w559) -> ("error out"=w551:errorcluster)  [unwired: 9 in, 1 out]
        n217 = call <vilib>:"IDtoNode.vi"("error in"=w551, "ID"=w560) -> ("error out"=w552:errorcluster, "invalid Id"=w555:bool, "node ref"=w554:T3)  [unwired: 7 in]
        n218 = case shown="False" w555 {
          tunnel: w554 -> [w567 _]
          tunnel: [w568 w571] -> w550
          tunnel: w552 -> [w565 w572]
          tunnel: w557 -> [w563 _]
          tunnel: w553 -> [w564 w569]
          tunnel: w549 -> [w561 w570]
          frame False {
            n219 = call "Remove UI without races.vi"("error in"=w565, "user event ref"=w564, "sub panel ref in"=w561) -> ("error out"=w566:errorcluster, "sub panel ref out"=w562:refnum<vi>)  [unwired: 7 in]
            n220 = call <vilib>:"LoadNodeUI.vi"("user event out"=w564, "error in"=w566, "sub panel ref in"=w562, "main queue"=w563, "node"=w567) -> ("error out"=w568:errorcluster)  [unwired: 6 in]
          }
          frame True {
            n221 = call "Remove UI without races.vi"("error in"=w572, "user event ref"=w569, "sub panel ref in"=w570) -> ("error out"=w571:errorcluster)  [unwired: 7 in, 1 out]
          }
        }
        n222 = call <vilib>:"Unset Busy.vi"("error in (no error)"=w550) -> ("error out"=w558:errorcluster)  [unwired: 10 in]
      }
      frame "Move" {
        n223 = Unflatten From String(type=T15 {"node ref"=refnum, "new parent"=refnum} ("Cluster"), binary string=w583, error in (no error)=w582) -> (value=w578:T15, error out=w577:errorcluster)  [unwired: 2 in, 1 out]
        n224 = Unbundle By Name(w578) -> ("node ref"=w574:T3, "new parent"=w573:T3)
        n225 = call <vilib>:"MoveNode.vi"("error in"=w577, "new parent"=w573, "node"=w574) -> ("error out"=w575:errorcluster)  [unwired: 8 in]
        n226 = call <vilib>:"Send Local Message.vi"("message queue in"=w580, "message name"="PopulateTree", "error in"=w575) -> ("error out"=w581:errorcluster)  [unwired: 10 in, 2 out]
      }
      frame "RefreshNodeView" {
        # "This user event is used by editor nodes to update their subpanels when data in the tree changes."
        n227 = Unbundle By Name(w586) -> ("user event ref"=w585:T4)
        n228 = Generate User Event(user event=w585, event data cluster=T8 {"command"="Refresh", "data"=""} ("event data"), error in=w588) -> (error out=w587:errorcluster)  [unwired: 1 in, 1 out]
      }
    }
  }
  n229 = while "User Interface Event Handler" {
    tunnel: w12 -> [w594]
    tunnel: w10 -> [w590]
    stop <- w593 stop-if-true
    n230 = event shown="[1] \"View\": Shortcut Menu Selection (User)" {
      selector: _ -> [_ _ _ _ _ _ _ _ _]
      dyn-events: _ -> [_ _ _ _ _ _ _ _ _]
      timeout: _ -> [_ _ _ _ _ _ _ _ _]
      tunnel: w594 -> [w602 w628 w670 w710 w717 w744 w748 w758 w763]
      tunnel: [_ _ _ TRUE _ _ _ _ _] -> w593
      tunnel: [w602 w620 w672 w706 w717 w741 w748 w756 w762] -> w592
      tunnel: [w597 w621 w671 w707 w713 w740 w745 w754 w760] -> w591
      tunnel: w590 -> [w601 w626 w669 w708 w716 w739 w747 w755 w761]
      event "View": Shortcut Menu Activation? {
        n231 = event-data() -> ("CtlRef"=w608:refnum<vi>, "Coords"=w607:T24, "MenuRef"=w604:refnum<k9>)  [unwired: 1 in]
        n232 = invoke class="Tree (strict)" method="Point To Row Column"(reference=w608, error in=w601, "Point"=w607) -> (error out=w600:errorcluster, "Tag"=w606:string)  [unwired: 5 in, 6 out]
        n233 = call <vilib>:"IDtoNode.vi"("error in"=w600, "ID"=w606) -> ("error out"=w598:errorcluster, "invalid Id"=w603:bool, "node ref"=w605:T3)  [unwired: 7 in]
        n234 = case shown="False" w603 {
          selector: w603 -> [_ w618]
          tunnel: w605 -> [w612 _]
          tunnel: w604 -> [w611 _]
          tunnel: [w610 _] -> w599
          tunnel: [w609 _] -> w596
          tunnel: [_ w618] -> w595
          frame False {
            n235 = in-place {
              in-place-border: w611 -> [w615]
              in-place-border: [w613] -> w610
              n236 = in-place-dvr #7(w612) -> (w617:refnum<class "NISE_CEF_Node.lvclass">, w614:errorcluster)
              n237 = call-dynamic "ShortcutMenu.vi"("error in"=w614, "menu ref in"=w615, "node in"=w617) -> ("error out"=w613:errorcluster, "node out"=w616:refnum<class "NISE_CEF_Node.lvclass">)  [unwired: 6 in, 1 out]
              n238 = in-place-dvr #7(w616) -> (w609:errorcluster)  [unwired: 1 out]
            }
          }
          frame True {
          }
        }
        n239 = Merge Errors(w596, w599, w598) -> (w597:errorcluster)
        n240 = event-data("Discard?"=w595) -> ()  [unwired: 1 in, 1 out]
      }
      event "View": Shortcut Menu Selection (User) {
        # "=nodeID"
        n241 = event-data() -> ("ItemPath"=w624:string, "CtlRef"=w631:refnum<vi>, "Coords"=w632:T24)  [unwired: 1 in]
        n242 = invoke class="Tree (strict)" method="Point To Row Column"(reference=w631, error in=w626, "Point"=w632) -> (error out=w625:errorcluster, "Tag"=w627:string)  [unwired: 5 in, 6 out]
        n243 = Match Pattern(string=w624, regular expression=":") -> (before substring=w630:string, after substring=w629:string)  [unwired: 1 in, 2 out]
        n244 = case shown="\"Add\"" w630 {
          tunnel: w629 -> [_ _ _ w661]
          tunnel: w628 -> [w639 w650 w656 w663]
          tunnel: w627 -> [w637 w644 w654 w662]
          tunnel: [w636 w648 w653 w659] -> w623
          tunnel: [w635 w647 w651 w657] -> w622
          tunnel: w625 -> [w634 w643 w652 w658]
          tunnel: w624 -> [_ w640 _ _]
          frame "Remove" {
            n245 = call <vilib>:"Send Local Message.vi"("message queue in"=w639, "message name"="RemoveNode" ("Message Name"), "message value"=w637, "error in"=w634) -> ("message queue out"=w636:T6, "error out"=w635:errorcluster)  [unwired: 9 in, 1 out]
          }
          frame Default {
            n246 = Bundle By Name(cluster=T13 {"node id"="", "RightClickPath"=""} ("input cluster"), "node id"=w644, "RightClickPath"=w640) -> (w645:T13)
            n247 = Flatten To String(anything=w645, error in (no error)=w643) -> (data string=w641:string, error out=w642:errorcluster)  [unwired: 2 in, 1 out]
            n248 = call <vilib>:"Send Local Message.vi"("message queue in"=w650, "message name"="HandleMenu" ("Message Name"), "message value"=w641, "error in"=w642) -> ("message queue out"=w648:T6, "error out"=w647:errorcluster)  [unwired: 9 in, 1 out]
          }
          frame "Duplicate" {
            n249 = call <vilib>:"Send Local Message.vi"("message queue in"=w656, "message name"="Duplicate" ("Message Name"), "message value"=w654, "error in"=w652) -> ("message queue out"=w653:T6, "error out"=w651:errorcluster)  [unwired: 9 in, 1 out]
          }
          frame "Add" {
            n250 = Bundle By Name(cluster=T14 {"node type"="", "to add to"=""} ("input cluster"), "node type"=w661, "to add to"=w662) -> (w664:T14)
            n251 = Flatten To String(anything=w664) -> (data string=w665:string)  [unwired: 3 in, 2 out]
            n252 = call <vilib>:"Send Local Message.vi"("message queue in"=w663, "message name"="AddNode" ("Message Name"), "message value"=w665, "error in"=w658) -> ("message queue out"=w659:T6, "error out"=w657:errorcluster)  [unwired: 9 in, 1 out]
          }
        }
        n253 = call <vilib>:"Send Local Message.vi"("message queue in"=w623, "message name"="RefreshNodeView", "error in"=w622) -> ("message queue out"=w620:T6, "error out"=w621:errorcluster)  [unwired: 10 in, 1 out]
      }
      event "View": Drop {
        n254 = event-data() -> ("CtlRef"=w668:refnum<vi>, "Coords"=w667:T24)  [unwired: 1 in]
        n255 = invoke class="Tree (strict)" method="Point To Row Column"(reference=w668, error in=w669, "Point"=w667) -> (reference out=w686:refnum<vi>, error out=w685:errorcluster, "Tag"=w682:string)  [unwired: 5 in, 5 out]
        n256 = call <vilib>:"ValidDragDrop.vi"("error in"=w685, "drag over"=w682, "tree ref in"=w686) -> ("error out"=w677:errorcluster, "accepted"=w680:bool, "drag"=w684:string, "tree ref out"=w687:refnum<vi>)  [unwired: 5 in]
        n257 = call <vilib>:"IDtoNode.vi"("error in"=w677, "ID"=w682) -> ("error out"=w678:errorcluster, "invalid Id"=w675:bool, "node ref"=w681:T3)  [unwired: 7 in]
        n258 = call <vilib>:"IDtoNode.vi"("error in"=w678, "ID"=w684) -> ("error out"=w676:errorcluster, "invalid Id"=w674:bool, "node ref"=w683:T3)  [unwired: 7 in]
        n259 = Compound Arithmetic op=AND(w680, invert w675, invert w674) -> (w679:bool)
        n260 = case shown="True" w679 {
          tunnel: w684 -> [_ w703]
          tunnel: w687 -> [_ w705]
          tunnel: [_ TRUE] -> w673
          tunnel: w682 -> [_ w701]
          tunnel: w670 -> [w689 w690]
          tunnel: [w689 w697] -> w672
          tunnel: [w688 w696] -> w671
          tunnel: w683 -> [_ w692]
          tunnel: w681 -> [_ w691]
          tunnel: w676 -> [w688 w693]
          frame False {
          }
          frame True {
            n261 = invoke class="Tree (strict)" method="Edit Tree Items.Move Item"(reference=w705, error in=w693, "tag"=w703, "New Parent"=w701) -> (error out=w694:errorcluster)  [unwired: 3 in, 6 out]
            n262 = Bundle By Name(cluster=T15 {"node ref"=refnum, "new parent"=refnum} ("Cluster"), "new parent"=w691, "node ref"=w692) -> (w700:T15)
            n263 = Flatten To String(anything=w700, error in (no error)=w694) -> (data string=w699:string, error out=w695:errorcluster)  [unwired: 2 in, 1 out]
            n264 = call <vilib>:"Send Local Message.vi"("message queue in"=w690, "message name"="Move", "message value"=w699, "error in"=w695) -> ("message queue out"=w697:T6, "error out"=w696:errorcluster)  [unwired: 9 in, 1 out]
          }
        }
        n265 = event-data("Accepted?"=w673) -> ()  [unwired: 1 in, 1 out]
      }
      event "Exit": Value Change {
        # "Exit the application                                           >> Stop this message generator loop    Cleaning errors if the other loop stop this one"
        n266 = event-data() -> ()  [unwired: 1 in, 1 out]
        n267 = call <vilib>:"Send Local Message.vi"("message queue in"=w710, "message name"="Close", "error in"=w708) -> ("message queue out"=w706:T6, "error out"=w711:errorcluster)  [unwired: 10 in, 1 out]
        n268 = call <vilib>:"Clear Errors.vi"("error in (no error)"=w711) -> ("error out"=w707:errorcluster)  [unwired: 6 in]
      }
      event "View": Drag Starting? {
        n269 = event-data() -> ("Data"=w723:T25, "CtlRef"=w725:refnum<vi>, "Coords"=w724:T24)  [unwired: 1 in]
        n270 = invoke class="Tree (strict)" method="Point To Row Column"(reference=w725, error in=w716, "Point"=w724) -> (error out=w715:errorcluster, "Tag"=w722:string)  [unwired: 5 in, 6 out]
        n271 = call <vilib>:"IDtoNode.vi"("error in"=w715, "ID"=w722) -> ("error out"=w714:errorcluster, "invalid Id"=w721:bool, "node ref"=w720:T3)  [unwired: 7 in]
        n272 = case shown="False" w721 {
          tunnel: w720 -> [w731 _]
          tunnel: [w728 TRUE ("Removable")] -> w718
          tunnel: w714 -> [w727 w737]
          tunnel: [w726 w737] -> w713
          frame False {
            n273 = in-place {
              in-place-border: [w734] -> w730
              in-place-border: w727 -> [w733]
              in-place-border: [w732] -> w726
              n274 = in-place-dvr #8(w731) -> (w736:refnum<class "NISE_CEF_Node.lvclass">)  [unwired: 1 out]
              n275 = call-dynamic "EditOptions.vi"("error in"=w733, "node in"=w736) -> ("error out"=w732:errorcluster, "edit options"=w734:T26, "node out"=w735:refnum<class "NISE_CEF_Node.lvclass">)  [unwired: 6 in, 1 out]
              n276 = in-place-dvr #8(w735) -> ()  [unwired: 2 out]
            }
            n277 = Unbundle By Name(w730) -> ("movable"=w729:bool)
            n278 = Not(x=w729) -> (.not. x?=w728:bool)
          }
          frame True {
          }
        }
        n279 = event-data("Data"=w723, "Drag Mode"=enum32{"copy or move", "copy only", "move only"}."move only", "Discard?"=w718) -> ()  [unwired: 1 in, 1 out]
      }
      event "View": Value Change {
        n280 = event-data() -> ("NewVal"=w742:string)  [unwired: 1 in]
        n281 = call <vilib>:"Send Local Message.vi"("message queue in"=w744, "message name"="ActivateNode" ("Message Name"), "message value"=w742, "error in"=w739) -> ("message queue out"=w741:T6, "error out"=w740:errorcluster)  [unwired: 9 in, 1 out]
      }
      event "View": event type 3.0.xa000003a {
        n282 = event-data() -> ("CtlRef"=w753:refnum<vi>, "Coords"=w750:T24)  [unwired: 1 in]
        n283 = invoke class="Tree (strict)" method="Point To Row Column"(reference=w753, error in=w747, "Point"=w750) -> (reference out=w752:refnum<vi>, error out=w746:errorcluster, "Tag"=w751:string)  [unwired: 5 in, 5 out]
        n284 = call <vilib>:"ValidDragDrop.vi"("error in"=w746, "drag over"=w751, "tree ref in"=w752) -> ("error out"=w745:errorcluster, "accepted"=w749:bool)  [unwired: 5 in, 2 out]
        n285 = event-data("Accepted?"=w749) -> ()  [unwired: 1 in, 1 out]
      }
      event Panel Close? {
        # "Intercepts the upper right close panel operation to allow a smooth shutdown as opposed to immediately killing the app."
        n286 = event-data() -> ()  [unwired: 1 in, 1 out]
        n287 = call <vilib>:"Send Local Message.vi"("message queue in"=w758, "message name"="Close?", "error in"=w755) -> ("message queue out"=w756:T6, "error out"=w754:errorcluster)  [unwired: 10 in, 1 out]
        n288 = event-data("Discard?"=TRUE) -> ()  [unwired: 1 in, 1 out]
      }
      event Menu Selection (User) {
        n289 = event-data() -> ("ItemPath"=w764:string)  [unwired: 1 in]
        n290 = case shown="\"_Tools:Save Binary\"" w764 {
          tunnel: w763 -> [w766 w772 w777 w782 w787 w792 w801 w806 w811 w816 w821 w827 w831]
          tunnel: [w766 w768 w773 w778 w783 w788 w798 w803 w808 w813 w818 w824 w830] -> w762
          tunnel: w761 -> [w765 w770 w775 w780 w785 w790 w797 w804 w809 w814 w819 w825 w829]
          tunnel: [w765 w769 w774 w779 w784 w789 w795 w802 w807 w812 w817 w823 w828] -> w760
          frame Default {
            n291 = One Button Dialog(message="Unknown Menu Option") -> ()  [unwired: 1 in, 1 out]
          }
          frame "_File:_New" {
            n292 = call <vilib>:"Send Local Message.vi"("message queue in"=w772, "message name"="New?" ("Message Name"), "error in"=w770) -> ("message queue out"=w768:T6, "error out"=w769:errorcluster)  [unwired: 10 in, 1 out]
          }
          frame "_File:_Open" {
            n293 = call <vilib>:"Send Local Message.vi"("message queue in"=w777, "message name"="Open?" ("Message Name"), "error in"=w775) -> ("message queue out"=w773:T6, "error out"=w774:errorcluster)  [unwired: 10 in, 1 out]
          }
          frame "_File:_Save" {
            n294 = call <vilib>:"Send Local Message.vi"("message queue in"=w782, "message name"="Save" ("Message Name"), "error in"=w780) -> ("message queue out"=w778:T6, "error out"=w779:errorcluster)  [unwired: 10 in, 1 out]
          }
          frame "_File:Save As..." {
            n295 = call <vilib>:"Send Local Message.vi"("message queue in"=w787, "message name"="SaveAs" ("Message Name"), "error in"=w785) -> ("message queue out"=w783:T6, "error out"=w784:errorcluster)  [unwired: 10 in, 1 out]
          }
          frame "_File:_Exit" {
            n296 = call <vilib>:"Send Local Message.vi"("message queue in"=w792, "message name"="Close?" ("Message Name"), "error in"=w790) -> ("message queue out"=w788:T6, "error out"=w789:errorcluster)  [unwired: 10 in, 1 out]
          }
          frame "_Tools:Multiple Parameter Editor" {
            n297 = call <vilib>:"Send Local Message.vi"("message queue in"=w801, "message name"="CleansubPanel", "error in"=w797) -> ("message queue out"=w800:T6, "error out"=w796:errorcluster)  [unwired: 10 in, 1 out]
            n298 = call <vilib>:"Send Local Message.vi"("message queue in"=w800, "message name"="Custom View", "message value"="Multiple Parameter Editor" ("Message Name"), "error in"=w796) -> ("message queue out"=w798:T6, "error out"=w795:errorcluster)  [unwired: 9 in, 1 out]
          }
          frame "_Tools:Test" {
            n299 = call <vilib>:"Send Local Message.vi"("message queue in"=w806, "message name"="Test", "error in"=w804) -> ("message queue out"=w803:T6, "error out"=w802:errorcluster)  [unwired: 10 in, 1 out]
          }
          frame "_Tools:Deploy Tool" {
            n300 = call <vilib>:"Send Local Message.vi"("message queue in"=w811, "message name"="DeployTool", "error in"=w809) -> ("message queue out"=w808:T6, "error out"=w807:errorcluster)  [unwired: 10 in, 1 out]
          }
          frame "_Tools:Save Binary" {
            n301 = call <vilib>:"Send Local Message.vi"("message queue in"=w816, "message name"="Save Binary", "error in"=w814) -> ("message queue out"=w813:T6, "error out"=w812:errorcluster)  [unwired: 10 in, 1 out]
          }
          frame "_Tools:Load Binary" {
            n302 = call <vilib>:"Send Local Message.vi"("message queue in"=w821, "message name"="Load Binary", "error in"=w819) -> ("message queue out"=w818:T6, "error out"=w817:errorcluster)  [unwired: 10 in, 1 out]
          }
          frame "_Tools:Refresh Plugins" {
            n303 = call <vilib>:"Send Local Message.vi"("message queue in"=w827, "message name"="FindPluginNodes", "message value"="Refresh", "error in"=w825) -> ("message queue out"=w824:T6, "error out"=w823:errorcluster)  [unwired: 9 in, 1 out]
          }
          frame "_Tools:Edit Plugin Search Paths" {
            n304 = call <vilib>:"Send Local Message.vi"("message queue in"=w831, "message name"="Edit Plugin Search Paths", "error in"=w829) -> ("message queue out"=w830:T6, "error out"=w828:errorcluster)  [unwired: 10 in, 1 out]
          }
        }
      }
    }
    n305 = call "send error message.vi"("error in"=w591, "message queue in"=w592) -> ()  [unwired: 9 in, 1 out]
  }
